vi "CreatePizza.vi"(8 "error in (no error)":errorcluster, 10 "Pizza to order":T1, 11 "NYPizzaStore in":refnum<class "NYPizzaStore.lvclass">) -> (0 "error out":errorcluster, 2 "Pizza object":refnum<class "Pizza.lvclass">, 3 "NYPizzaStore out":refnum<class "NYPizzaStore.lvclass">)   [LabVIEW 2021, in "NYPizzaStore.lvclass"]
uses:
  NYPizzaStore.lvclass
  Pizza/pizza types.ctl
  Pizza/Pizza.lvclass
  NYStyleCheesePizza/NYStyleCheesePizza.lvclass
  C:/Users/nina/Documents/Head First Design Patterns/HeadFirstDesignPatternsLabVIEWandPython/04 Factory/LabVIEW/Pizza/Pizza.lvclass
  NYStylePepperoniPizza/NYStylePepperoniPizza.lvclass
panel:
  # "Connector Pane"
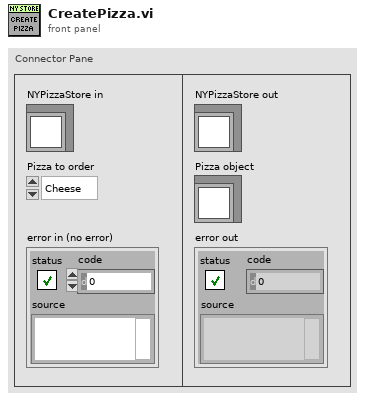
[diagram p1: front panel]
types:
  T1 = typedef "Pizza.lvclass/pizza types.ctl" = enum16{"Cheese", "Pepperoni"}
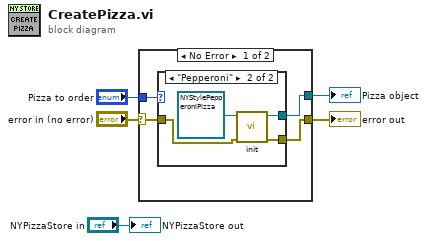
[diagram p0: block diagram]
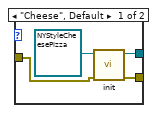
[diagram p2: hidden frame]
diagram:
  n1 = case shown="No Error" "error in (no error)" {
    selector: "error in (no error)" -> [w7 w18]
    tunnel: "Pizza to order" -> [w9 _]
    tunnel: [w8 _] -> w2
    tunnel: [w6 w18] -> w1
    frame No Error {
      n2 = case shown="\"Pepperoni\"" w9 {
        tunnel: [w10 w16] -> w8
        tunnel: w7 -> [w12 w14]
        tunnel: [w11 w15] -> w6
        frame "Cheese", Default {
          n3 = call "init.vi"("error in (no error)"=w12, "NYStyleCheesePizza in"=refnum<class "NYStyleCheesePizza.lvclass"> refnum ("NYStyleCheesePizza.lvclass")) -> ("error out"=w11:errorcluster, "NYStyleCheesePizza out"=w10:refnum<class "NYStyleCheesePizza.lvclass">)  [unwired: 8 in]
        }
        frame "Pepperoni" {
          n4 = call "init.vi"("error in (no error)"=w14, "NYStyleCheesePizza in"=refnum<class "NYStylePepperoniPizza.lvclass"> refnum ("NYStylePepperoniPizza.lvclass")) -> ("error out"=w15:errorcluster, "NYStyleCheesePizza out"=w16:refnum<class "NYStylePepperoniPizza.lvclass">)  [unwired: 8 in]
        }
      }
    }
    frame Error {
    }
  }
  "error out" <- w1
  "Pizza object" <- w2
  "NYPizzaStore out" <- "NYPizzaStore in"
